vi "Start Stream VCam.vi"(7 "Correlation ID":u32, 8 "error in (no error)":errorcluster, 10 "Camera Settings":T1={"Exposure Time (ms)"=100.0, "Binning"=enum."2x2", "Scan Mode"=0, "Frames to Acquire"=1000.0, "Pixel Correction"=FALSE, "Frames to Skip"=0, "File Path"=path "", "Duty cycle"=0.0, "ALEX"=FALSE, "Shutter Enable"=[], "fluidics trigger, ms (0=disabled)"=0.0, "Bit Depth"=16, "Image Width (px)"=0, "Image Height (px)"=0, "Horizontal Offset (px)"=0, "Vertical Offset (px)"=0} {"fluidics trigger, ms (0=disabled)" max=60000.0 step=1.0; "Exposure Time (ms)" min=1.0 max=10000.0 step=1.0}, 11 "Application in":refnum<class "Application.lvclass">) -> (0 "error out":errorcluster, 2 "Success?":bool, 3 "Application out":refnum<class "Application.lvclass">)   [LabVIEW 2023, in "Application.lvlib" / "Application.lvclass"]
uses:
  Application.lvclass
  Resources/Type Defs/Camera Settings.ctl
  Application.lvclass/Application.ctl
  Hardware/Device Messages/Save CorrID Msg/Save CorrID Msg.lvclass/Save CorrID Msg.ctl
  <vilib>/ActorFramework/Message Enqueuer/Message Enqueuer.lvclass/Message Enqueuer.ctl
  Hardware/Camera Messages/Start Stream Msg/Start Stream Msg.lvclass/Start Stream Msg.ctl
  <vilib>/ActorFramework/Message Enqueuer/Enqueue.vi
  Hardware/Device Messages/Save CorrID Msg/Save CorrID Msg.lvclass
  C:/Program Files/National Instruments/LabVIEW 2023/vi.lib/ActorFramework/Message/Message.lvclass
  Hardware/Camera Messages/Start Stream Msg/Start Stream Msg.lvclass
  Resources/GLOBAL/GLOBAL Time-critical.vi
  <vilib>/ActorFramework/Message Priority Queue/Priority Enqueue.vi
  Application.lvlib
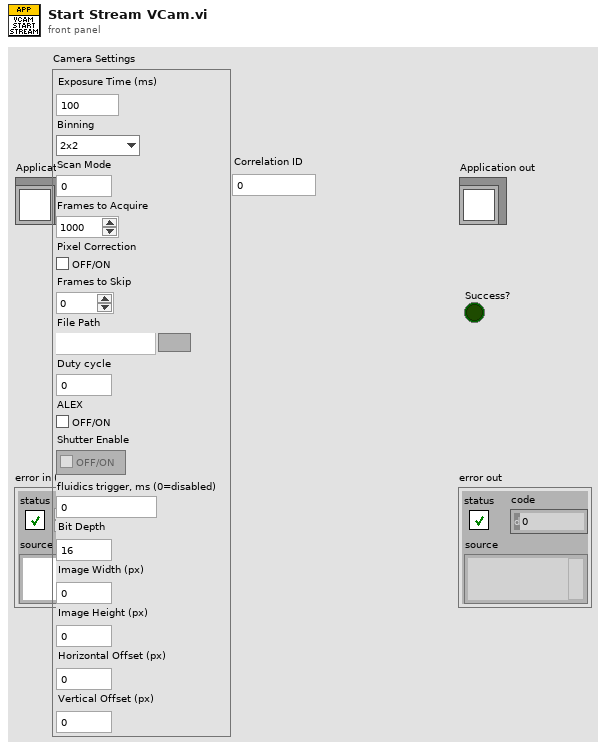
[diagram p1: front panel]
types:
  T1 = typedef "Camera Settings.ctl" = cluster{"Exposure Time (ms)":dbl, "Binning":enum16{"1x1", "2x2", "4x4"}, "Scan Mode":i32, "Frames to Acquire":dbl, "Pixel Correction":bool, "Frames to Skip":u32, "File Path":path, "Duty cycle":dbl, "ALEX":bool, "Shutter Enable":bool[], "fluidics trigger, ms (0=disabled)":dbl, "Bit Depth":u16, "Image Width (px)":u16, "Image Height (px)":u16, "Horizontal Offset (px)":u16, "Vertical Offset (px)":u16}
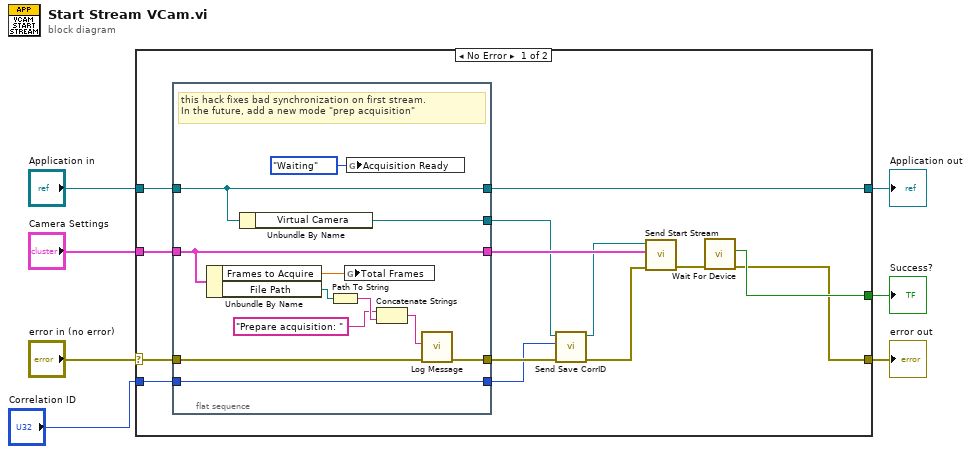
[diagram p0: block diagram]
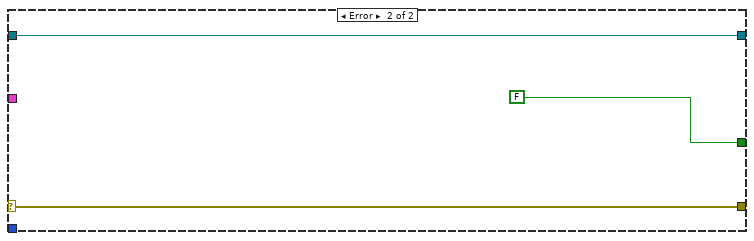
[diagram p2: hidden frame]
diagram:
  n1 = case shown="No Error" "error in (no error)" {
    selector: "error in (no error)" -> [w15 w36]
    tunnel: [w8 w36] -> w6
    tunnel: [w20 w35] -> w4
    tunnel: "Application in" -> [w21 w35]
    tunnel: "Camera Settings" -> [w19 _]
    tunnel: [w16 FALSE ("Success?")] -> w2
    tunnel: "Correlation ID" -> [w14 _]
    frame No Error {
      n2 = flat-sequence {
        tunnel: w21 -> [w33]
        tunnel: [w33] -> w20
        tunnel: w19 -> [w31]
        tunnel: [w31] -> w18
        tunnel: w15 -> [w29]
        tunnel: [w28] -> w13
        tunnel: [w27] -> w11
        tunnel: w14 -> [w22]
        tunnel: [w22] -> w9
        frame #0 {
          # "this hack fixes bad synchronization on first stream.\nIn the future, add a new mode \"prep acquisition\""
          n3 = Unbundle By Name(w31) -> ("Frames to Acquire"=w32:dbl, "File Path"=w26:path)
          n4 = Unbundle By Name(w33) -> ("Virtual Camera"=w27:refnum<class "Message Enqueuer.lvclass">)
          n5 = Path To String(path=w26) -> (string=w25:string)
          n6 = global write "GLOBAL Time-critical.vi" "Total Frames"(w32) -> ()
          n7 = global write "GLOBAL Time-critical.vi" "Acquisition Ready"(enum16{"Waiting", "Ready", "Fail", "Timeout"}."Waiting" ("Acquisition Ready")) -> ()
          n8 = Concatenate Strings("Prepare acquisition: " ("input"), w25) -> (w23:string)
          n9 = call "Log Message.vi"("error constant"=w29, "input"=w23) -> ("error constant 2"=w28:errorcluster)  [unwired: 8 in, 1 out]
        }
      }
      n10 = call "Send Save CorrID.vi"("error in (no error)"=w13, "Correlation ID"=w9, "Message Enqueuer"=w11) -> ("error out"=w12:errorcluster, "Message Enqueuer out"=w10:refnum<class "Message Enqueuer.lvclass">)  [unwired: 7 in]
      n11 = call "Send Start Stream.vi"("error in (no error)"=w12, "Camera Settings"=w18, "Message Enqueuer"=w10) -> ("error out"=w17:errorcluster)  [unwired: 7 in, 1 out]
      n12 = call "Wait For Device.vi"("error in"=w17) -> ("error out"=w8:errorcluster, "Success?"=w16:bool)  [unwired: 9 in]
    }
    frame Error {
    }
  }
  "error out" <- w6
  "Application out" <- w4
  "Success?" <- w2
